vi "__keysight_t2_measurement_(Multi_pulse_Keysight_AWG_T2_two_volatile).vi"() -> ()   [LabVIEW 2013]
uses:
  <vilib>/Analysis/baseanly.llb/Mean (DBL).vi
  <vilib>/Analysis/NI_AALBase.lvlib
  <instrlib>/Rohde&Schwarz Vector Network Analyzer/Rohde&Schwarz Vector Network Analyzer.lvlib
panel:
  out "Keysight settings":T1 {"Frequency 1 (Hz)" format="%#_6p"; "Frequency 2 (Hz)" format="%#_6p"}
  out "Total time between P1 and Bucket (ns)":i32
  out "Current spacing (ns)":i32
  in  "Gen Power dBm":dbl=10.0 caption="Gen Power, dBm" format="%#.3f"
  in  "Gen Freq:":dbl=8880700000.0 format="%^#.6e"
  out "Points per ns":i32
  in  "N-per-period":i32=20001
  in  "Keysight Period (ns)":u16=3 max=15
  out "Bucket width (points)":i32
  out "Moovie":dbl[][](graph)
  out "Real":dbl[](graph)=[4.942129453411326e-05, 4.669294139603153e-05, 4.9292413677903824e-05, 4.8073251491587143e-05]
  out "Imaginary":dbl[](graph)
  in  "VNA Power dBm":dbl=-15.0 caption="VNA Power, dBm" format="%#.3f"
  in  "Center Freq:":dbl=6092900000.0 format="%^#.6e"
  in  "Span Freq:":dbl=10000.0 format="%^#.3e"
  in  "Bandwidth:":dbl=1.0 caption="Bandwidth (1 to 1e6 Hz):" format="%#.3f"
  in  "Points:":i32=4
  in  "Sweep Type":i32(ring)=4 caption="Sweep Type:" items=["Lin. Frequency", "Log. Frequency", "Segmented Frequency", "Power", "CW Mode", "Time"]
  out "No of Values":i32
  in  "Train Width 3 (ns)":i32
  in  "Train Width 2 (ns)":i32
  in  "Train Width 1 (ns)":i32
  in  "Train offset (ns)":i32
  in  "Bucket offset (ns)":i32
  in  "Steps size (ns)":i32
  in  "Steps":i32
  in  "Bucket Width (ns)":i32=20001
  in  "Connection":T2={"Type"=1, "VISA"="TCPIP0::192.168.0.8::inst0::INSTR", "GPIB"="10"} {"Type" items=["VISA", "GPIB"]}
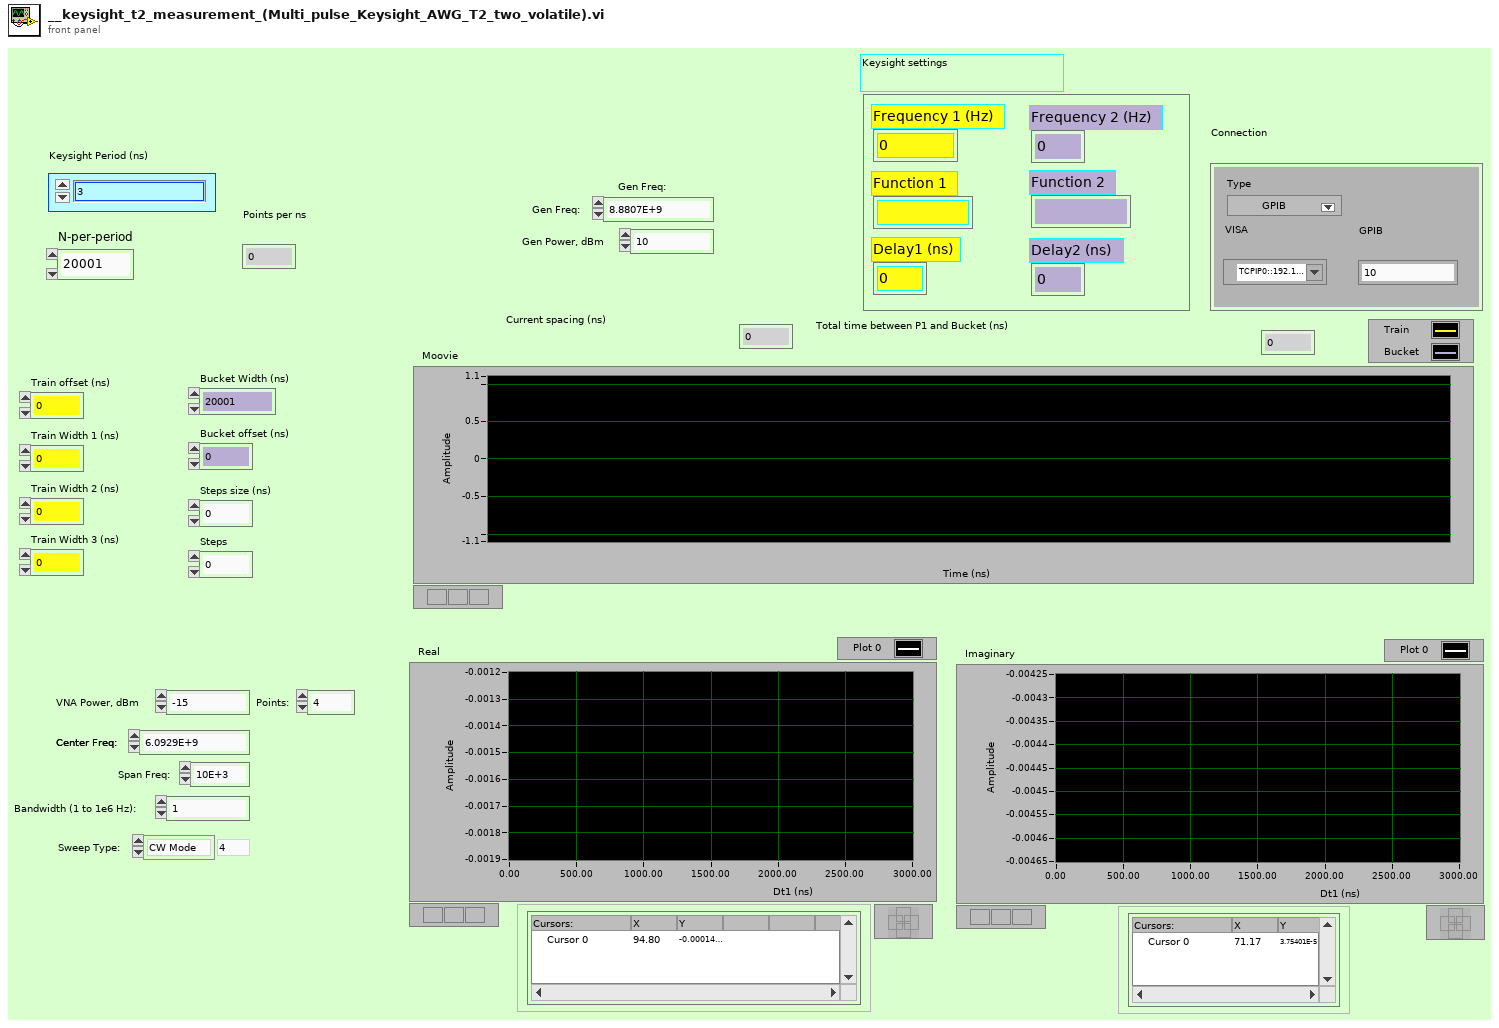
[diagram p1: front panel]
types:
  T1 = cluster{"Frequency 2 (Hz)":dbl, "Function 2":string, "Delay2 (ns) ":dbl, "Frequency 1 (Hz)":dbl, "Function 1":string, "Delay1 (ns)":dbl}
  T2 = cluster{"Type":u16, "VISA":refnum<visa-resource-name>, "GPIB":string}
  T3 = cluster{"Coupling":bool, "Frequency 2 (MHz)":dbl, "Frequency 1 (MHz)":dbl, "WAVEFORM":enum32{"PULSE", "ARBITRARY"}}
  T4 = cluster{"Ouput 1":bool, "Ouput 2":bool, "Ouput 1 Neg":bool, "Ouput 2 Neg":bool}
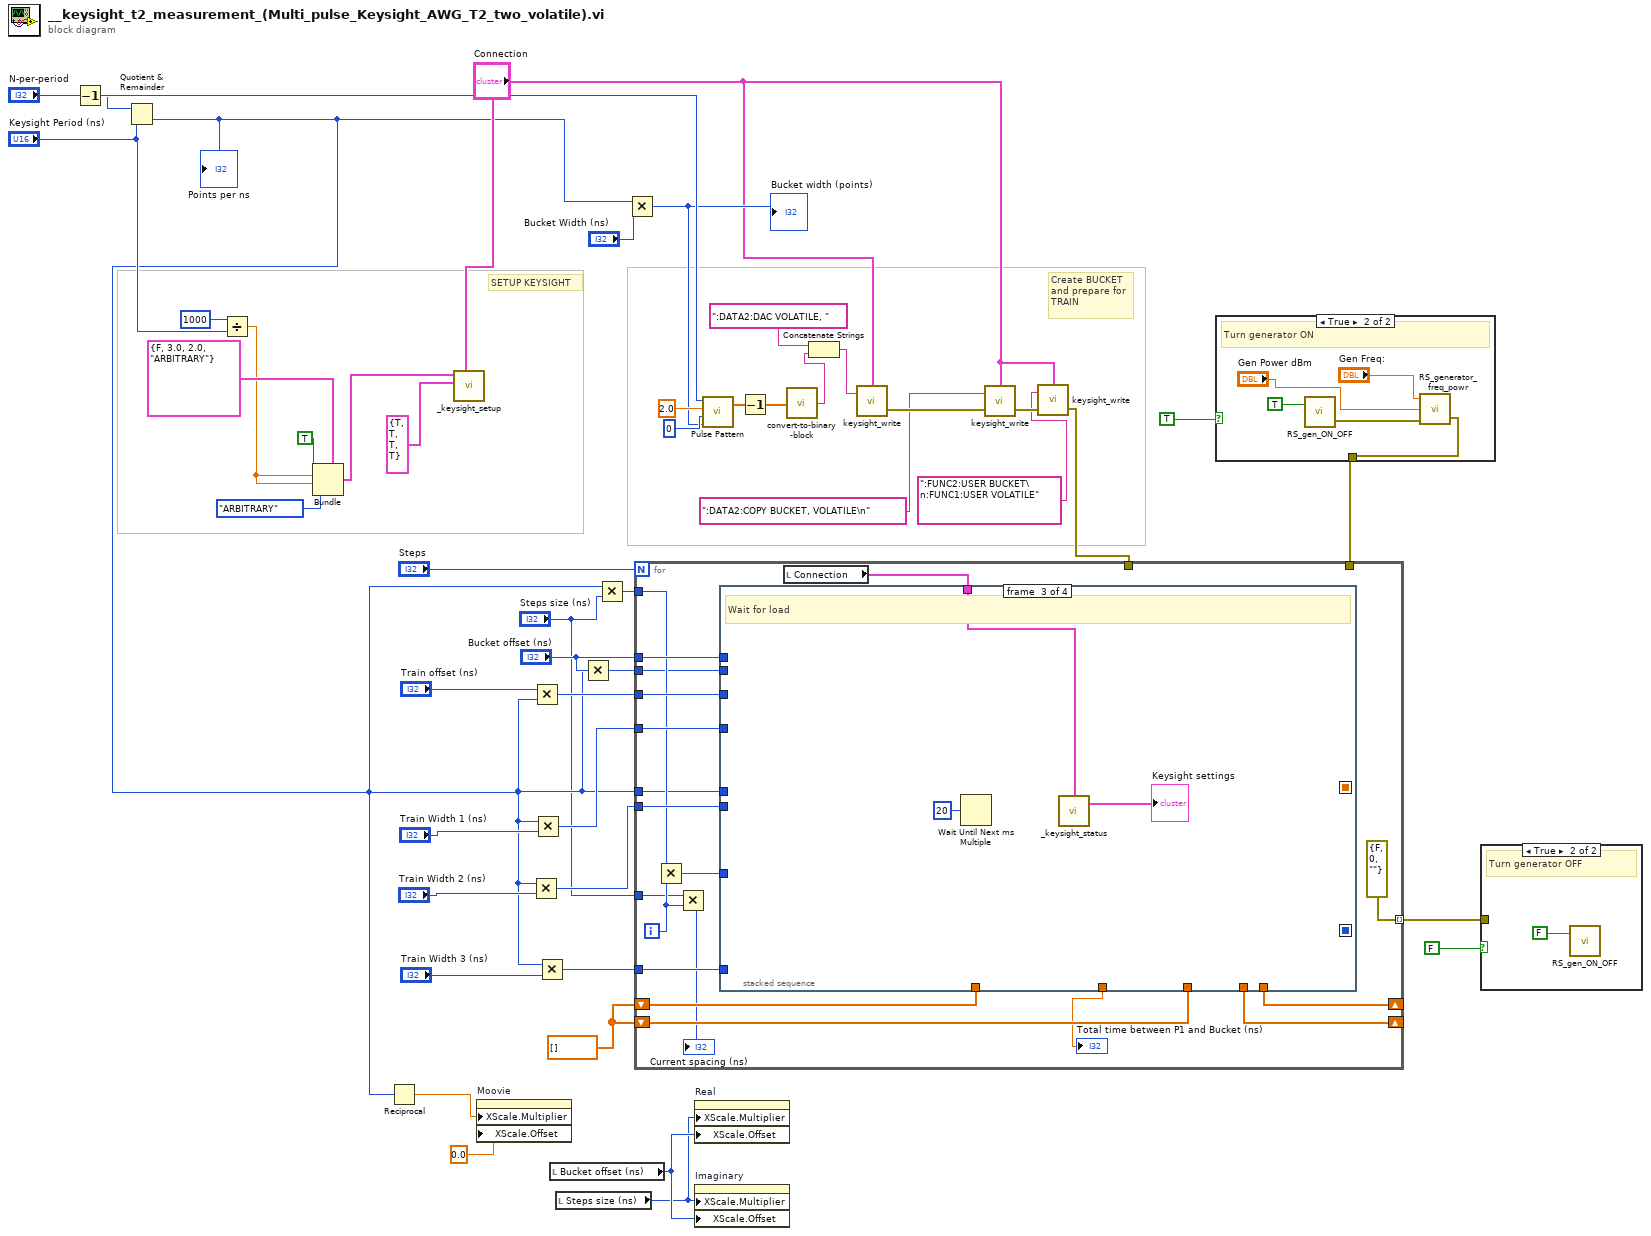
[diagram p0: block diagram]
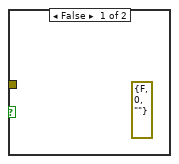
[diagram p2: hidden frame]
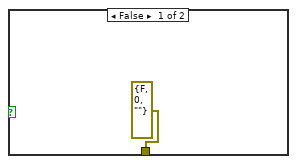
[diagram p3: hidden frame]
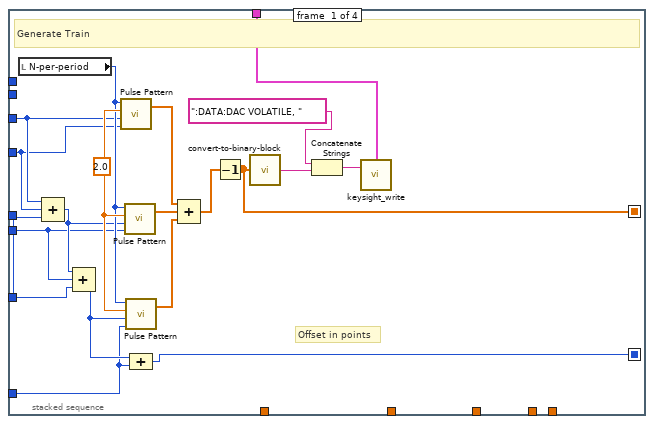
[diagram p4: hidden frame]
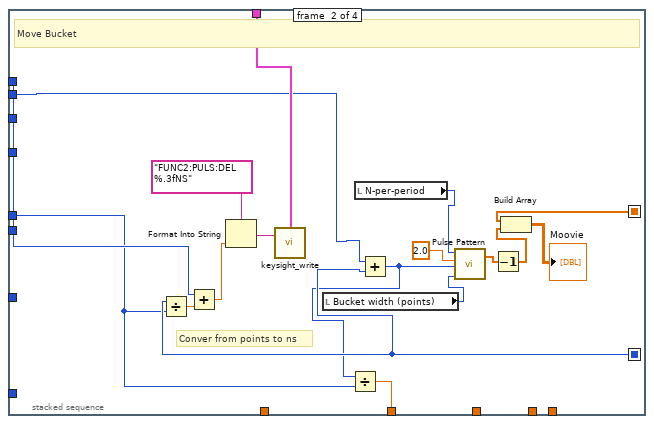
[diagram p5: hidden frame]
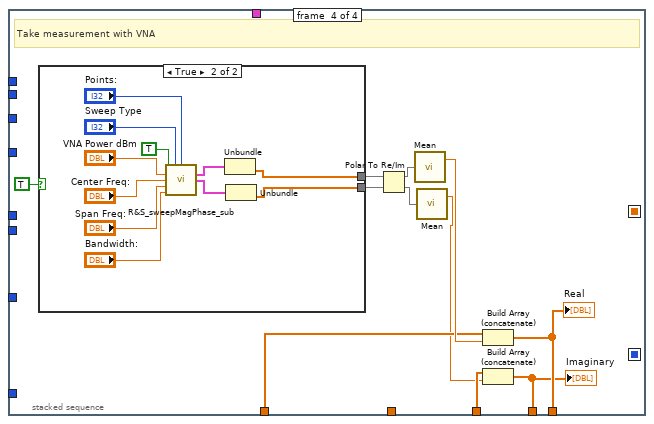
[diagram p6: hidden frame]
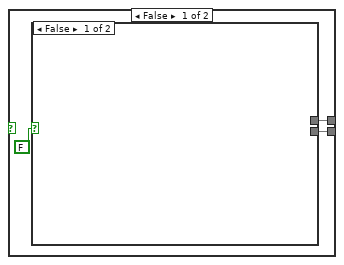
[diagram p7: hidden frame]
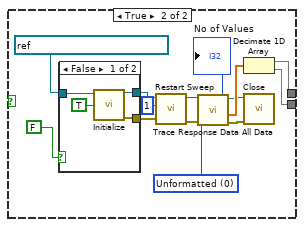
[diagram p8: hidden frame]
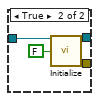
[diagram p9: hidden frame]
diagram:
  w19 = dbl[] []
  # "Create BUCKET\nand prepare for\nTRAIN"
  # "SETUP KEYSIGHT"
  n1 = Decrement(x="N-per-period") -> (x-1=w33:i32)
  n2 = Quotient & Remainder(x=w33, y="Keysight Period (ns)") -> (floor(x/y)=w4:i32)  [unwired: 1 out]
  "Points per ns" <- w4
  n3 = Divide(x=u16 1000, y="Keysight Period (ns)") -> (x/y=w35:dbl)
  n4 = Bundle(cluster=T3 {"Coupling"=FALSE, "Frequency 2 (MHz)"=3.0, "Frequency 1 (MHz)"=2.0, "WAVEFORM"=enum."ARBITRARY"} ("Frequency Parameters"), "Coupling"=TRUE, "Frequency 2 (MHz)"=w35, "Frequency 1 (MHz)"=w35, "WAVEFORM"=enum32{"PULSE", "ARBITRARY"}."ARBITRARY") -> (w44:T3)
  n5 = Reciprocal(x=w4) -> (1/x=w14:dbl)
  n6 = call "_keysight_setup.vi"("Frequency Parameters"=w44, "Outputs"=T4 {"Ouput 1"=TRUE, "Ouput 2"=TRUE, "Ouput 1 Neg"=TRUE, "Ouput 2 Neg"=TRUE}, "Connection"="Connection") -> ()  [unwired: 3 in, 1 out]
  n7 = property on="Moovie" class="WFGraph (strict)"("XScale.Multiplier"=w14, "XScale.Offset"=0.0 ("X Scale.Offset and Multiplier:Offset")) -> ()  [unwired: 2 in, 2 out]
  n8 = Multiply(x=w4, y="Train Width 2 (ns)") -> (x*y=w22:i32)
  n9 = Multiply(x="Train offset (ns)", y=w4) -> (x*y=w23:i32)
  n10 = Multiply(x=w4, y="Train Width 1 (ns)") -> (x*y=w25:i32)
  n11 = Multiply(x=w4, y="Train Width 3 (ns)") -> (x*y=w20:i32)
  n12 = local read "Bucket offset (ns)"() -> (w13:i32)
  n13 = local read "Steps size (ns)"() -> (w12:i32)
  n14 = Multiply(x="Bucket offset (ns)", y=w4) -> (x*y=w3:i32)
  n15 = Multiply(x=w4, y="Steps size (ns)") -> (x*y=w21:i32)
  n16 = Multiply(x=w4, y="Bucket Width (ns)") -> (x*y=w30:i32)
  "Bucket width (points)" <- w30
  n17 = property on="Real" class="WFGraph (strict)"("XScale.Multiplier"=w12, "XScale.Offset"=w13) -> ()  [unwired: 2 in, 2 out]
  n18 = property on="Imaginary" class="WFGraph (strict)"("XScale.Multiplier"=w12, "XScale.Offset"=w13) -> ()  [unwired: 2 in, 2 out]
  n19 = call <vilib>:"Pulse Pattern.vi"("width"=w30, "delay"=0, "amplitude"=2.0, "samples"="N-per-period") -> ("Pulse Pattern"=w11:dbl[])  [unwired: 1 out]
  n20 = Decrement(x=w11) -> (x-1=w10:dbl[])
  n21 = call "convert-to-binary-block.vi"("Array to Binary Block Format"=w10) -> ("Binary Block"=w40:string)
  n22 = Concatenate Strings(":DATA2:DAC VOLATILE, ", w40) -> (w39:string)
  n23 = call "keysight_write.vi"("command"=w39, "Connection"="Connection") -> ("error out"=w38:errorcluster)  [unwired: 2 in]
  n24 = call "keysight_write.vi"("error in"=w38, "command"=":DATA2:COPY BUCKET, VOLATILE\n", "Connection"="Connection") -> ("error out"=w9:errorcluster)  [unwired: 1 in]
  n25 = call "keysight_write.vi"("error in"=w9, "command"=":FUNC2:USER BUCKET\n:FUNC1:USER VOLATILE", "Connection"="Connection") -> ("error out"=w8:errorcluster)  [unwired: 1 in]
  n26 = case shown="True" TRUE {
    tunnel: [errorcluster {"status"=FALSE, "code"=0, "source"=""} ("error out") w52] -> w2
    frame False {
    }
    frame True {
      # "Turn generator ON"
      n27 = call "RS_gen_ON_OFF.vi"("Generator Output"=TRUE) -> ("error out"=w53:errorcluster)  [unwired: 1 in]
      n28 = call "RS_generator_freq_powr.vi"("error in"=w53, "Power (dBm)"="Gen Power dBm", "Frequnecy (Hz)"="Gen Freq:") -> ("error out"=w52:errorcluster)  [unwired: 1 out]
    }
  }
  n29 = for {
    N: "Steps" -> [_]
    tunnel: "Bucket offset (ns)" -> [w73]
    tunnel: w8 -> [_]
    tunnel: w25 -> [w71]
    tunnel: w23 -> [w70]
    tunnel: w22 -> [w69]
    tunnel: w21 -> [w68]
    tunnel: w20 -> [w67]
    shift-right: [w63] -> _
    shift-left: w19 -> [w64]
    shift-right: [w65] -> _
    shift-left: w19 -> [w66]
    tunnel: w2 -> [_]
    tunnel: [errorcluster {"status"=FALSE, "code"=0, "source"=""} ("error out")] -> w16 mode=indexing
    tunnel: w4 -> [w59]
    tunnel: w3 -> [w61]
    tunnel: "Steps size (ns)" -> [w56]
    i -> [w57]
    n30 = Multiply(x=w68, y=w57) -> (x*y=w60:i32)
    n31 = Multiply(x=w56, y=w57) -> (x*y=→"Current spacing (ns)":i32)
    n32 = local read "Connection"() -> (w72:T2)
    n33 = stacked-sequence {
      seq-local: [w76 _ _ _] -> [_ w96 _ _]
      seq-local: [w74 _ _ _] -> [_ w101 _ _]
      tunnel: w73 -> [_ w106 _ _]
      tunnel: w72 -> [w84 w108 w112 _]
      tunnel: w71 -> [w82 _ _ _]
      tunnel: w70 -> [w83 _ _ _]
      tunnel: w69 -> [w80 _ _ _]
      tunnel: w60 -> [w79 _ _ _]
      tunnel: w67 -> [w77 _ _ _]
      tunnel: w66 -> [_ _ _ w116]
      tunnel: [_ _ _ w119] -> w65
      tunnel: w64 -> [_ _ _ w115]
      tunnel: [_ _ _ w118] -> w63
      tunnel: w59 -> [_ w94 _ _]
      tunnel: w61 -> [_ w97 _ _]
      tunnel: [_ w93 _ _] -> w55
      frame #0 {
        w92 = 2.0 ("amplitude")
        # "Offset in points"
        # "Generate Train"
        n34 = local read "N-per-period"() -> (w91:i32)
        n35 = Compound Arithmetic op=ADD(w83, w82, w79) -> (w81:i32)
        n36 = Compound Arithmetic op=ADD(w81, w80, w79) -> (w78:i32)
        n37 = call <vilib>:"Pulse Pattern.vi"("width"=w82, "delay"=w83, "amplitude"=w92, "samples"=w91) -> ("Pulse Pattern"=w90:dbl[])  [unwired: 1 out]
        n38 = call <vilib>:"Pulse Pattern.vi"("width"=w80, "delay"=w81, "amplitude"=w92, "samples"=w91) -> ("Pulse Pattern"=w89:dbl[])  [unwired: 1 out]
        n39 = call <vilib>:"Pulse Pattern.vi"("width"=w77, "delay"=w78, "amplitude"=w92, "samples"=w91) -> ("Pulse Pattern"=w88:dbl[])  [unwired: 1 out]
        n40 = Compound Arithmetic op=ADD(w78, w77) -> (w76:i32)
        n41 = Compound Arithmetic op=ADD(w90, w89, w88) -> (w75:dbl[])
        n42 = Decrement(x=w75) -> (x-1=w74:dbl[])
        n43 = call "convert-to-binary-block.vi"("Array to Binary Block Format"=w74) -> ("Binary Block"=w86:string)
        n44 = Concatenate Strings(":DATA:DAC VOLATILE, ", w86) -> (w85:string)
        n45 = call "keysight_write.vi"("command"=w85, "Connection"=w84) -> ()  [unwired: 2 in, 1 out]
      }
      frame #1 {
        # "Conver from points to ns"
        # "Move Bucket"
        n46 = Divide(x=w96, y=w94) -> (x/y=w107:dbl)
        n47 = Add(x=w106, y=w107) -> (x+y=w105:dbl)
        n48 = Format Into String(format string="FUNC2:PULS:DEL %.3fNS", w105) -> (resulting string=w109:string)  [unwired: 2 in, 1 out]
        n49 = call "keysight_write.vi"("command"=w109, "Connection"=w108) -> ()  [unwired: 2 in, 1 out]
        n50 = local read "Bucket width (points)"() -> (w103:i32)
        n51 = local read "N-per-period"() -> (w98:i32)
        n52 = Add(x=w97, y=w96) -> (x+y=w95:i32)
        n53 = Divide(x=w95, y=w94) -> (x/y=w93:dbl)
        n54 = call <vilib>:"Pulse Pattern.vi"("width"=w103, "delay"=w95, "amplitude"=2.0, "samples"=w98) -> ("Pulse Pattern"=w102:dbl[])  [unwired: 1 out]
        n55 = Decrement(x=w102) -> (x-1=w99:dbl[])
        n56 = Build Array(w101, w99) -> (→"Moovie":dbl[][])
      }
      frame #2 {
        # "Wait for load"
        n57 = Wait Until Next ms Multiple(millisecond multiple=u32 20) -> ()  [unwired: 1 out]
        n58 = call "_keysight_status.vi"("Connection"=w112) -> ("Keysight settings"=→"Keysight settings":T1)  [unwired: 2 in, 1 out]
      }
      frame #3 {
        # "Take measurement with VNA"
        n59 = case shown="True" TRUE {
          tunnel: [w127 w150] -> w121
          tunnel: [w126 w151] -> w120
          frame False {
            n60 = case shown="False" FALSE {
              tunnel: [_ w135] -> w127
              tunnel: [_ w134] -> w126
              frame False {
              }
              frame True {
                w140 = 0 items=["Unformatted", "Formatted", "Unformatted With Trace Mathematics"] ("Data Format (Unformatted)")
                n61 = case shown="False" FALSE ("Boolean") {
                  tunnel: [w142 w149] -> w131
                  tunnel: [w143 w148] -> w133
                  tunnel: refnum<visa-resource-name> "TCPIP::192.168.0.3::INST" ("VISA resource name") -> [w144 w147]
                  frame False {
                    n62 = call <instrlib>:"Initialize.vi"("VISA resource name"=w144, "Reset (T: Reset)"=TRUE) -> ("VISA resource name out"=w143:refnum<visa-resource-name>, "error out"=w142:errorcluster)  [unwired: 12 in]
                  }
                  frame True {
                    n63 = call <instrlib>:"Initialize.vi"("VISA resource name"=w147, "Reset (T: Reset)"=FALSE) -> ("VISA resource name out"=w148:refnum<visa-resource-name>, "error out"=w149:errorcluster)  [unwired: 12 in]
                  }
                }
                n64 = call <instrlib>:"Restart Sweep.vi"("error in (no error)"=w131, "Channel (1)"=1, "VISA resource name"=w133) -> ("error out"=w130:errorcluster, "VISA resource name out"=w132:refnum<visa-resource-name>)  [unwired: 7 in]
                n65 = call <instrlib>:"Trace Response Data All Data.vi"("error in (no error)"=w130, "Data Format (Unformatted)"=w140, "VISA resource name"=w132) -> ("error out"=w139:errorcluster, "Trace Data"=w141:dbl[], "No of Values"=→"No of Values":i32, "VISA resource name out"=w138:refnum<visa-resource-name>)  [unwired: 5 in]
                n66 = Decimate 1D Array(w141) -> (w135:dbl[], w134:dbl[])
                n67 = call <instrlib>:"Close.vi"("error in (no error)"=w139, "VISA resource name"=w138) -> ()  [unwired: 9 in, 1 out]
              }
            }
          }
          frame True {
            n68 = call "R&S_sweepMagPhase_sub.vi"("Boolean"=TRUE, "Sweep Type"="Sweep Type", "Points:"="Points:", "Power dBm"="VNA Power dBm", "Center Freq:"="Center Freq:", "Span Freq:"="Span Freq:", "Bandwidth:"="Bandwidth:") -> ("Lin Mag"=w152:cluster{dbl[], dbl[]}, "Phase"=w153:cluster{dbl[], dbl[]})  [unwired: 7 in]
            n69 = Unbundle(w152) -> (w150:dbl[])  [unwired: 1 out]
            n70 = Unbundle(w153) -> (w151:dbl[])  [unwired: 1 out]
          }
        }
        n71 = Polar To Re/Im(2:w120, 3:w121) -> (0:w122:dbl[], 1:w123:dbl[])
        n72 = call-poly <vilib>:"Mean.vi"("X"=w123) -> ("mean"=w117:dbl)  [unwired: 1 out]
        n73 = call-poly <vilib>:"Mean.vi"("X"=w122) -> ("mean"=w114:dbl)  [unwired: 1 out]
        n74 = Build Array (concatenate)(w116, w117) -> (w119:dbl[])
        "Real" <- w119
        n75 = Build Array (concatenate)(w115, w114) -> (w118:dbl[])
        "Imaginary" <- w118
      }
    }
    "Total time between P1 and Bucket (ns)" <- w55
  }
  n76 = case shown="True" FALSE {
    tunnel: w16 -> [_ _]
    frame False {
      (unwired) errorcluster {"status"=FALSE, "code"=0, "source"=""} ("error out")
    }
    frame True {
      # "Turn generator OFF"
      n77 = call "RS_gen_ON_OFF.vi"("Generator Output"=FALSE) -> ()  [unwired: 1 in, 1 out]
    }
  }
